vi "CRYFlatten Curve Test Info.vi"(11 "unflattened test info data":cluster{"Original Res":string, "Steps":i32}) -> (3 "Flattened Data":string)   [LabVIEW 2013]
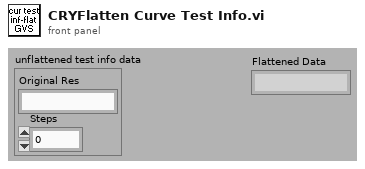
[diagram p1: front panel]
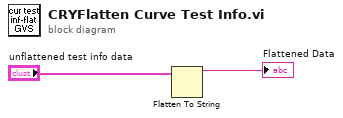
[diagram p0: block diagram]
diagram:
  n1 = Flatten To String(anything="unflattened test info data") -> (data string=→"Flattened Data":string)  [unwired: 1 in, 4 out]
